vi "TrajectoryCreateExecuteAbsolute.vi"(8 "Init":bool, 11 "End Pose ENG":T1={"TRANSLATION"={"X"=0.0, "Y"=0.0}, "ROTATION"={"VALUE"=0.0, "COS"=1.0, "SIN"=0.0}} {"ROTATION"."SIN" format="%13.4f"; "ROTATION"."COS" format="%13.4f"; "ROTATION"."VALUE" format="%13.4f"; "TRANSLATION"."Y" format="%14.3f"; "TRANSLATION"."X" format="%14.3f"}) -> (0 "AtReference":bool, 3 "Chassis Velocity Target":T4 {"vOmega" format="%10.3f"; "vY" format="%10.3f"; "vX" format="%10.3f"})   [LabVIEW 2023]
uses:
  <vilib>/Rock Robotics/WPI/ThirdParty/JAS_Junk/TrajLib/TypeDef/CHASSIS_SPEEDS.ctl
  <vilib>/Rock Robotics/WPI/ThirdParty/JAS_Junk/TrajLib/TypeDef/POSE2D.ctl
  <vilib>/Rock Robotics/WPI/ThirdParty/JAS_Junk/TrajLib/TypeDef/TRANSLATION2D.ctl
  <vilib>/Rock Robotics/WPI/ThirdParty/JAS_Junk/TrajLib/TypeDef/ROTATION2D.ctl
  <vilib>/Rock Robotics/WPI/ThirdParty/JAS_Junk/TrajLib/VI/Util_GetTime_U32.vi
  <vilib>/Rock Robotics/WPI/ThirdParty/JAS_Junk/TrajLib/HolDrvCtrl_New.vi
  <vilib>/Rock Robotics/WPI/ThirdParty/JAS_Junk/TrajLib/HolDrvCtrl_PackPID.vi
  <vilib>/Rock Robotics/WPI/ThirdParty/JAS_Junk/TrajLib/HolDrvCtrl_SetTolerance.vi
  <vilib>/Rock Robotics/WPI/ThirdParty/JAS_Junk/TrajLib/HolDrvCtrl_SetEnabled.vi
  <vilib>/Rock Robotics/WPI/ThirdParty/JAS_Junk/TrajLib/HolDrvCtrl_Calculate_Trajectory.vi
  <vilib>/Rock Robotics/WPI/ThirdParty/JAS_Junk/TrajLib/HolDrvCtrl_AtReference.vi
  <vilib>/Rock Robotics/WPI/ThirdParty/JAS_Junk/TrajLib/ProfiledPIDController_NewPeriod.vi
  <vilib>/Rock Robotics/WPI/ThirdParty/JAS_Junk/TrajLib/ProfiledPIDController_SetIntegratorRange.vi
  <vilib>/Rock Robotics/WPI/ThirdParty/JAS_Junk/TrajLib/ProfiledPIDController_DisableContInput.vi
  <vilib>/Rock Robotics/WPI/ThirdParty/JAS_Junk/TrajLib/ProfiledPIDController_EnableContInput.vi
  <vilib>/Rock Robotics/WPI/ThirdParty/JAS_Junk/TrajLib/TrapProfConstraint_New.vi
  <vilib>/Rock Robotics/WPI/ThirdParty/JAS_Junk/TrajLib/Rotation2d_CreateAngle.vi
  <vilib>/Rock Robotics/WPI/ThirdParty/JAS_Junk/TrajLib/Translation2d_Create.vi
  <vilib>/Rock Robotics/WPI/ThirdParty/JAS_Junk/TrajLib/Conv_Deg_Radians.vi
  <vilib>/Rock Robotics/WPI/ThirdParty/JAS_Junk/TrajLib/PIDController_NewPeriod.vi
  <vilib>/Rock Robotics/WPI/ThirdParty/JAS_Junk/TrajLib/PIDController_SetIntegratorRange.vi
  <vilib>/Rock Robotics/WPI/ThirdParty/JAS_Junk/TrajLib/PIDController_Reset.vi
  <vilib>/Rock Robotics/WPI/ThirdParty/JAS_Junk/TrajLib/HolDrvCtrl_Calculate.vi
  <vilib>/Rock Robotics/WPI/ThirdParty/JAS_Junk/TrajLib/Rotation2d_GetRadians.vi
  <vilib>/Rock Robotics/WPI/ThirdParty/JAS_Junk/TrajLib/TrapProfState_New.vi
  <vilib>/Rock Robotics/SystemInterfaces/NetworkCommunication/NetComm_UsageReport_report.vi
  <vilib>/Rock Robotics/WPI/ThirdParty/JAS_Junk/TrajLib/PIDController_DisableContinousInput.vi
  <vilib>/Rock Robotics/WPI/ThirdParty/JAS_Junk/TrajLib/PIDController_EnableContinousInput.vi
  <vilib>/Rock Robotics/WPI/ThirdParty/JAS_Junk/TrajLib/Rotation2d_GetAngleCosSin.vi
  <vilib>/Rock Robotics/WPI/ThirdParty/JAS_Junk/TrajLib/Pose2d_RelativeTo.vi
  <vilib>/Rock Robotics/WPI/ThirdParty/JAS_Junk/TrajLib/Pose2d_getRotation.vi
  <vilib>/Rock Robotics/WPI/ThirdParty/JAS_Junk/TrajLib/Rotation2d_Minus.vi
  <vilib>/Rock Robotics/WPI/ThirdParty/JAS_Junk/TrajLib/ProfiledPIDController_Calculate_Meas_Goal.vi
  <vilib>/Rock Robotics/WPI/ThirdParty/JAS_Junk/TrajLib/PIDController_Calculate_SP_PV.vi
  <vilib>/Rock Robotics/WPI/ThirdParty/JAS_Junk/TrajLib/ProfiledPIDController_Reset_PosOnly.vi
  <vilib>/Rock Robotics/WPI/ThirdParty/JAS_Junk/TrajLib/ChassisSpeeds_FromFieldRelativeSpeeds.vi
  <vilib>/Rock Robotics/WPI/ThirdParty/JAS_Junk/TrajLib/Transform2d_Create_PosePose.vi
  <vilib>/Rock Robotics/WPI/ThirdParty/JAS_Junk/TrajLib/Pose2d_New_TRRO.vi
  <vilib>/Rock Robotics/WPI/ThirdParty/JAS_Junk/TrajLib/Rotation2d_UnaryMinus.vi
  <vilib>/Rock Robotics/WPI/ThirdParty/JAS_Junk/TrajLib/Rotation2d_RotateBy.vi
  <vilib>/Rock Robotics/WPI/ThirdParty/JAS_Junk/TrajLib/ProfiledPIDController_SetGoal_PosOnly.vi
  <vilib>/Rock Robotics/WPI/ThirdParty/JAS_Junk/TrajLib/ProfiledPIDController_Calculate_Meas.vi
  <vilib>/Rock Robotics/WPI/ThirdParty/JAS_Junk/TrajLib/PIDController_SetSetpoint.vi
  <vilib>/Rock Robotics/WPI/ThirdParty/JAS_Junk/TrajLib/PIDController_Calculate_PV.vi
  <vilib>/Rock Robotics/WPI/ThirdParty/JAS_Junk/TrajLib/ProfiledPIDController_Reset.vi
  <vilib>/Rock Robotics/WPI/ThirdParty/JAS_Junk/TrajLib/Rotation2d_GetCos.vi
  <vilib>/Rock Robotics/WPI/ThirdParty/JAS_Junk/TrajLib/Rotation2d_GetSin.vi
  <vilib>/Rock Robotics/WPI/ThirdParty/JAS_Junk/TrajLib/Translation2d_RotateBy.vi
  <vilib>/Rock Robotics/WPI/ThirdParty/JAS_Junk/TrajLib/Translation2d_Minus.vi
  <vilib>/Rock Robotics/WPI/ThirdParty/JAS_Junk/TrajLib/Rotation2d_CreateXY.vi
  <vilib>/Rock Robotics/WPI/ThirdParty/JAS_Junk/TrajLib/ProfiledPIDController_SetGoal.vi
  <vilib>/Rock Robotics/WPI/ThirdParty/JAS_Junk/TrajLib/TrapProfile_New.vi
  <vilib>/Rock Robotics/WPI/ThirdParty/JAS_Junk/TrajLib/ProfiledPIDController_GetPeriod.vi
  <vilib>/Rock Robotics/WPI/ThirdParty/JAS_Junk/TrajLib/TrapProfile_Calculate.vi
  <vilib>/Rock Robotics/WPI/ThirdParty/JAS_Junk/TrajLib/ControllerUtil_GetModulusError.vi
  <vilib>/Rock Robotics/WPI/ThirdParty/JAS_Junk/TrajLib/Util_CalcDist.vi
  <vilib>/Rock Robotics/WPI/ThirdParty/JAS_Junk/TrajLib/TrapProfile_ShouldFlipAcceleration.vi
  <vilib>/Rock Robotics/WPI/ThirdParty/JAS_Junk/TrajLib/TrapProfile_Direct.vi
  <vilib>/Rock Robotics/WPI/ThirdParty/JAS_Junk/TrajLib/PIDController_GetPeriod.vi
  Vision/VisionGlobal.vi
  TrajectoryGlobals.vi
  <vilib>/Rock Robotics/SystemInterfaces/Utilities/FPGA_UtilitiesRead LocalTime.vi
  <vilib>/Rock Robotics/WPI/ThirdParty/JAS_Junk/TrajLib/VI/Util_GetTime_U64.vi
  <vilib>/Rock Robotics/WPI/ThirdParty/JAS_Junk/TrajLib/Globals/Util_LibraryGlobals.vi
  <vilib>/Rock Robotics/WPI/ThirdParty/JAS_Junk/TrajLib/Trajectory_Library.lvlib
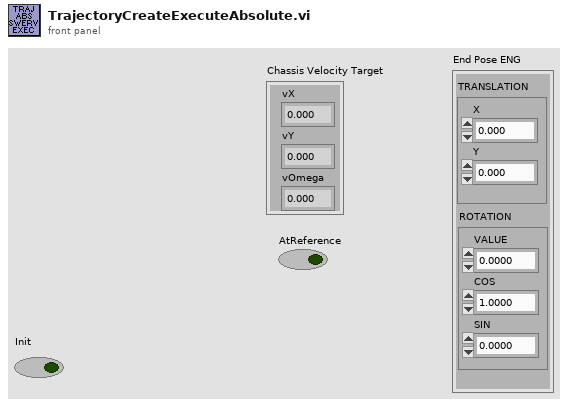
[diagram p1: front panel]
types:
  T1 = typedef "Trajectory_Library.lvlib/POSE2D.ctl" = cluster{"TRANSLATION":T2, "ROTATION":T3}
  T2 = typedef "Trajectory_Library.lvlib/TRANSLATION2D.ctl" = cluster{"X":dbl, "Y":dbl}
  T3 = typedef "Trajectory_Library.lvlib/ROTATION2D.ctl" = cluster{"VALUE":dbl, "COS":dbl, "SIN":dbl}
  T4 = typedef "Trajectory_Library.lvlib/CHASSIS_SPEEDS.ctl" = cluster{"vX":dbl, "vY":dbl, "vOmega":dbl}
  T5 = typedef "Trajectory_Library.lvlib/SWERVE_DRIVE_KINEMATICS.ctl" = cluster{"NumModules":i32, "InverseKinematics":T6, "ForwardKinematics":T6, "Modules":T2[], "PrevCoR":T2, "SavedModuleStates":T7[]}
  T6 = typedef "NI_Matrix.lvlib/RealMatrix.ctl" = dbl[][]
  T7 = typedef "Trajectory_Library.lvlib/SWERVE_DRIVE_MODULE_STATE.ctl" = cluster{"Speed":dbl, "Angle":T3}
  T8 = typedef "Trajectory_Library.lvlib/TRAJECTORY.ctl" = cluster{"TotalTImeSecs":dbl, "States":T9[]}
  T9 = typedef "Trajectory_Library.lvlib/TRAJ_STATE.ctl" = cluster{"TimeSeconds":dbl, "Velocity":dbl, "Acceleration":dbl, "POSE":T1, "Curvature":dbl}
  T10 = typedef "Trajectory_Library.lvlib/PID_TUNING.ctl" = cluster{"Kp":dbl, "Ki":dbl, "Kd":dbl, "MaximumIntegral":dbl, "MinimumIntegral":dbl, "IntegralZone":dbl}
  T11 = typedef "Trajectory_Library.lvlib/PROFILED_PID_CONTROLLER.ctl" = cluster{"Controller":T12, "Goal":T13, "Setpoint":T13, "Constraint":T14}
  T12 = typedef "Trajectory_Library.lvlib/PID_CONTROLLER.ctl" = cluster{"Kp":dbl, "Ki":dbl, "Kd":dbl, "Period":dbl, "Max_Integral":dbl, "Min_Integral":dbl, "Max_Input":dbl, "Min_Input":dbl, "Continuous":bool, "PositionError":dbl, "VelocityError":dbl, "PrevError":dbl, "Total_Integral":dbl, "PositionTolerance":dbl, "VelocityTolerance":dbl, "SetPoint":dbl, "Kf":dbl, "Prev_Deriv":dbl, "Prev_Deriv 2":dbl, "DerivativeFilter":bool, "Min_Output":dbl, "Max_Output":dbl, "Prev_F_P":dbl, "Prev_F_P_2":dbl, "AntiWindupActive":bool, "Measurement":dbl, "IntegralZone":dbl}
  T13 = typedef "Trajectory_Library.lvlib/TRAPEZOID_PROFILE_STATE.ctl" = cluster{"Position":dbl, "Velocity":dbl}
  T14 = typedef "Trajectory_Library.lvlib/TRAPEZOID_PROFILE_CONSTRAINT.ctl" = cluster{"MaxVelocity":dbl, "MaxAcceleration":dbl}
  T15 = typedef "Trajectory_Library.lvlib/HOLONOMIC_PACK_TUNING.ctl" = cluster{"X PID Tuning":T10, "Y PID Tuning":T10, "thetaProfiledPID_CTRL":T11}
  T16 = typedef "Trajectory_Library.lvlib/HOLONOMIC_DRV_CTRL.ctl" = cluster{"poseTolerance":T1, "poseError":T1, "Enabled":bool, "PID_xCtrl":T12, "PID_yCtrl":T12, "PROF_PID_thetaCtrl":T11, "RotationError":T3, "FirstRun":bool}
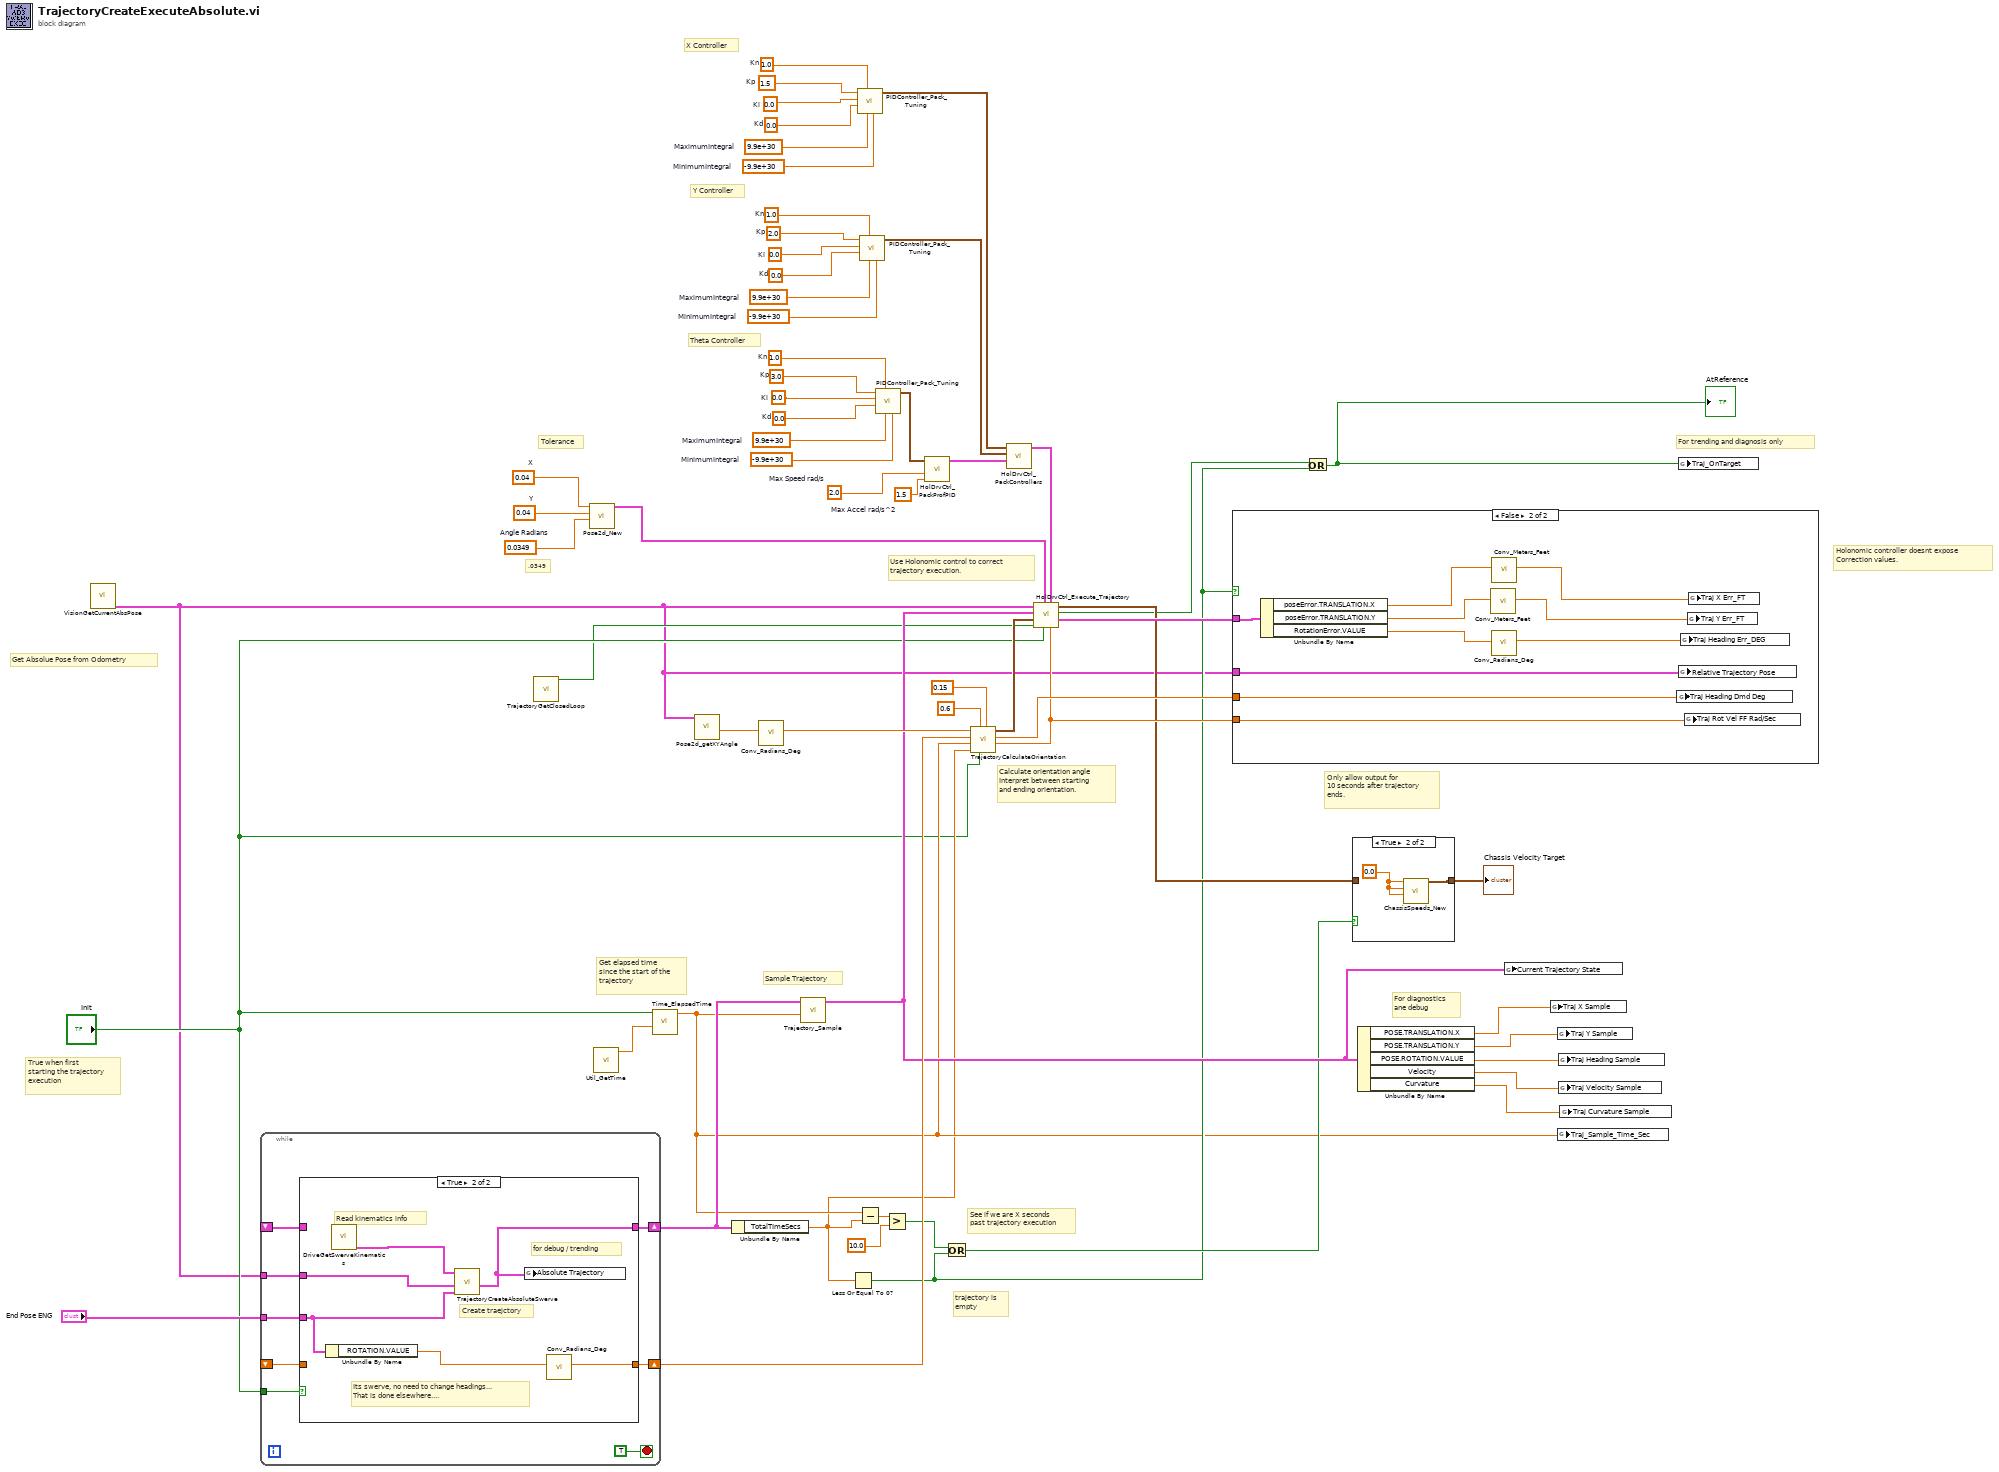
[diagram p0: block diagram]
diagram:
  w5 = 0.04  # X
  w4 = 0.04  # Y
  w6 = 0.0349  # Angle Radians
  w7 = 1.5  # Max Accel rad/s^2
  w8 = 2.0  # Max Speed rad/s
  w32 = 1.0  # Kn
  w35 = 3.0  # Kp
  w44 = 0.0  # Ki
  w45 = 0.0  # Kd
  w46 = 9.9e+30  # MaximumIntegral
  w47 = -9.9e+30  # MinimumIntegral
  w30 = 1.0  # Kn
  w33 = 1.5  # Kp
  w36 = 0.0  # Ki
  w37 = 0.0  # Kd
  w38 = 9.9e+30  # MaximumIntegral
  w39 = -9.9e+30  # MinimumIntegral
  w31 = 1.0  # Kn
  w34 = 2.0  # Kp
  w40 = 0.0  # Ki
  w41 = 0.0  # Kd
  w42 = 9.9e+30  # MaximumIntegral
  w43 = -9.9e+30  # MinimumIntegral
  # ".0349"
  # "Tolerance"
  # "trajectory is \nempty"
  # "Theta Controller"
  # "Y Controller"
  # "X Controller"
  # "Calculate orientation angle\nInterpret between starting\nand ending orientation."
  # "True when first\nstarting the trajectory\nexecution"
  # "Get elapsed time\nsince the start of the\ntrajectory"
  # "Holonomic controller doesnt expose\nCorrection values."
  # "Use Holonomic control to correct\ntrajectory execution."
  # "For trending and diagnosis only"
  # "For diagnostics\nane debug"
  # "Get Absolue Pose from Odometry"
  # "Sample Trajectory"
  # "See if we are X seconds \npast trajectory execution"
  # "Only allow output for\n10 seconds after trajectory\nends."
  n1 = call "VisionGetCurrentAbsPose.vi"() -> ("Current ABS Pose"=w9:T1)  [unwired: 9 in]
  n2 = while {
    tunnel: "Init" -> [w68]
    tunnel: w9 -> [w67]
    shift-right: [w66] -> w25
    shift-left: _ -> [w65]
    shift-right: [w64] -> w22
    shift-left: _ -> [w63]
    tunnel: "End Pose ENG" -> [w62]
    stop <- TRUE stop-if-true
    n3 = case shown="True" w68 {
      tunnel: w67 -> [_ w73]
      tunnel: [w71 w74] -> w66
      tunnel: w65 -> [w71 _]
      tunnel: [w70 w76] -> w64
      tunnel: w63 -> [w70 _]
      tunnel: w62 -> [_ w77]
      frame False {
      }
      frame True {
        # "for debug / trending"
        # "Read kinematics info"
        # "Its swerve, no need to change headings...\nThat is done elsewhere...."
        # "Create traejctory"
        n4 = Unbundle By Name(w77) -> ("ROTATION.VALUE"=w75:dbl)
        n5 = call "DriveGetSwerveKinematics.vi"() -> ("SWERVE_DRIVE_KINEMATICS"=w72:T5)  [unwired: 11 in]
        n6 = call "TrajectoryCreateAbsoluteSwerve.vi"("End Pose  ENG"=w77, "Current Pose SI"=w73, "SWERVE_DRIVE_KINEMATICS"=w72) -> ("Absolute Trajectory"=w74:T8)  [unwired: 6 in, 2 out]
        n7 = global write "TrajectoryGlobals.vi" "Absolute Trajectory"(w74) -> ()
        n8 = call <vilib>:"Conv_Radians_Deg.vi"("Radians"=w75) -> ("Degrees"=w76:dbl)  [unwired: 10 in]
      }
    }
  }
  n9 = call "TrajectoryGetClosedLoop.vi"() -> ("AUTO_CLOSED_LOOP"=w10:bool)  [unwired: 11 in]
  n10 = call <vilib>:"Pose2d_New.vi"("Heading"=w6, "Y"=w4, "X"=w5) -> ("out POSe"=w3:T1)  [unwired: 8 in]
  n11 = call <vilib>:"Util_GetTime.vi"() -> ("FPGA_Time_Seconds"=w58:dbl)  [unwired: 9 in, 2 out]
  n12 = call <vilib>:"Time_ElapsedTime.vi"("PassthroughTime_SEC"=w58, "Reset"="Init") -> ("Elapsed Time Sec"=w13:dbl)  [unwired: 9 in]
  n13 = call <vilib>:"Pose2d_getXYAngle.vi"("in POSE"=w9) -> ("Angle"=w24:dbl)  [unwired: 8 in, 2 out]
  n14 = Unbundle By Name(w25) -> ("TotalTImeSecs"=w12:dbl)
  n15 = call <vilib>:"Conv_Radians_Deg.vi"("Radians"=w24) -> ("Degrees"=w23:dbl)  [unwired: 10 in]
  n16 = call <vilib>:"Trajectory_Sample.vi"("Time"=w13, "InputTRAJECTORY"=w25) -> ("OutputTRAJ_STATE"=w21:T9)  [unwired: 9 in]
  n17 = Less Or Equal To 0?(x=w12) -> (x <= 0?=w14:bool)
  n18 = call <vilib>:"PIDController_Pack_Tuning.vi"("MinimumIntegral"=w39, "MaximumIntegral"=w38, "Kn"=w30, "Kd"=w37, "Ki"=w36, "Kp"=w33) -> ("PID Tuning"=w48:T10)  [unwired: 5 in]
  n19 = Subtract(x=w13, y=w12) -> (x-y=w61:dbl)
  n20 = call <vilib>:"PIDController_Pack_Tuning.vi"("MinimumIntegral"=w43, "MaximumIntegral"=w42, "Kn"=w31, "Kd"=w41, "Ki"=w40, "Kp"=w34) -> ("PID Tuning"=w49:T10)  [unwired: 5 in]
  n21 = call <vilib>:"PIDController_Pack_Tuning.vi"("MinimumIntegral"=w47, "MaximumIntegral"=w46, "Kn"=w32, "Kd"=w45, "Ki"=w44, "Kp"=w35) -> ("PID Tuning"=w29:T10)  [unwired: 5 in]
  n22 = Greater?(x=w61, y=10.0) -> (0:w18:bool)
  n23 = call <vilib>:"HolDrvCtrl_PackProfPID.vi"("Max Accel"=w7, "Max Speed"=w8, "Theta PID Tuning"=w29) -> ("Theta PID CONTROLLER"=w50:T11)  [unwired: 8 in]
  n24 = Or(x=w18, y=w14) -> (x .or. y?=w17:bool)
  n25 = call "TrajectoryCalculateOrientation.vi"("Starting Fraction"=0.15, "Init"="Init", "Completion Fraction"=0.6, "Total Trajectory Time Sec"=w12, "Elapsed Traj Time Sec"=w13, "End Orientation Demand DEG"=w22, "Starting Orientation  DEG"=w23) -> ("Rotational Velocity Rad Per Sec"=w26:dbl, "Orientation Demand Deg"=w52:dbl, "Orientation Demand"=w28:T3)  [unwired: 2 in]
  n26 = call <vilib>:"HolDrvCtrl_PackControllers.vi"("thetaProfiledPID_CTRL"=w50, "Y PID Tuning"=w49, "X PID Tuning"=w48) -> ("HOLONOMIC_CTRL_PACK_TUNING"=w51:T15)  [unwired: 8 in]
  n27 = call <vilib>:"HolDrvCtrl_Execute_Trajectory.vi"("Rotational Velocity Feedforward \nRad/Sec"=w26, "HOLONOMIC_CTRL_PACK_TUNING"=w51, "Reset"="Init", "Tolerance"=w3, "Enable"=w10, "angleRef"=w28, "desiredTrajState"=w21, "currentPose"=w9) -> ("outHOLONOMIC_DRV_CTRL"=w27:T16, "AtReference"=w16:bool, "calcChassisSpeed"=w19:T4)  [unwired: 1 in]
  n28 = case shown="False" w14 {
    tunnel: w52 -> [_ w87]
    tunnel: w27 -> [_ w81]
    tunnel: w26 -> [_ w80]
    tunnel: w9 -> [_ w78]
    frame True {
    }
    frame False {
      n29 = Unbundle By Name(w81) -> ("poseError.TRANSLATION.X"=w85:dbl, "poseError.TRANSLATION.Y"=w84:dbl, "RotationError.VALUE"=w79:dbl)
      n30 = call <vilib>:"Conv_Meters_Feet.vi"("Meters"=w84) -> ("Feet"=w83:dbl)  [unwired: 10 in]
      n31 = call <vilib>:"Conv_Radians_Deg.vi"("Radians"=w79) -> ("Degrees"=w86:dbl)  [unwired: 10 in]
      n32 = call <vilib>:"Conv_Meters_Feet.vi"("Meters"=w85) -> ("Feet"=w82:dbl)  [unwired: 10 in]
      n33 = global write "TrajectoryGlobals.vi" "Traj Heading Dmd Deg"(w87) -> ()
      n34 = global write "TrajectoryGlobals.vi" "Relative Trajectory Pose"(w78) -> ()
      n35 = global write "TrajectoryGlobals.vi" "Traj Heading Err_DEG"(w86) -> ()
      n36 = global write "TrajectoryGlobals.vi" "Traj Rot Vel FF Rad/Sec"(w80) -> ()
      n37 = global write "TrajectoryGlobals.vi" "Traj Y Err_FT"(w83) -> ()
      n38 = global write "TrajectoryGlobals.vi" "Traj X Err_FT"(w82) -> ()
    }
  }
  n39 = Or(x=w16, y=w14) -> (x .or. y?=w15:bool)
  "AtReference" <- w15
  n40 = case shown="True" w17 {
    tunnel: w19 -> [w88 _]
    tunnel: [w88 w89] -> w59
    frame False {
    }
    frame True {
      w90 = 0.0 ("vX")
      n41 = call <vilib>:"ChassisSpeeds_New.vi"("vAngular"=w90, "vY"=w90, "vX"=w90) -> ("CHASSIS"=w89:T4)  [unwired: 8 in]
    }
  }
  "Chassis Velocity Target" <- w59
  n42 = Unbundle By Name(w21) -> ("POSE.TRANSLATION.X"=w57:dbl, "POSE.TRANSLATION.Y"=w56:dbl, "POSE.ROTATION.VALUE"=w55:dbl, "Velocity"=w54:dbl, "Curvature"=w53:dbl)
  n43 = global write "TrajectoryGlobals.vi" "Current Trajectory State"(w21) -> ()
  n44 = global write "TrajectoryGlobals.vi" "Traj X Sample"(w57) -> ()
  n45 = global write "TrajectoryGlobals.vi" "Traj Y Sample"(w56) -> ()
  n46 = global write "TrajectoryGlobals.vi" "Traj_Sample_Time_Sec"(w13) -> ()
  n47 = global write "TrajectoryGlobals.vi" "Traj Heading Sample"(w55) -> ()
  n48 = global write "TrajectoryGlobals.vi" "Traj Velocity Sample"(w54) -> ()
  n49 = global write "TrajectoryGlobals.vi" "Traj Curvature Sample"(w53) -> ()
  n50 = global write "TrajectoryGlobals.vi" "Traj_OnTarget"(w15) -> ()
